vi "Calc Record Length.vi"(8 "error in (no error)":errorcluster, 11 "Modbus PLC in":refnum<class "Modbus PLC.lvclass">) -> (0 "error out":errorcluster, 3 "Modbus PLC out":refnum<class "Modbus PLC.lvclass">)   [LabVIEW 2023, in "Modbus PLC.lvlib" / "Modbus PLC.lvclass"]
uses:
  Modbus PLC.lvclass
  Modbus PLC.lvclass/Modbus PLC.ctl
panel:
  out "Array":i32[][](array[numeric])
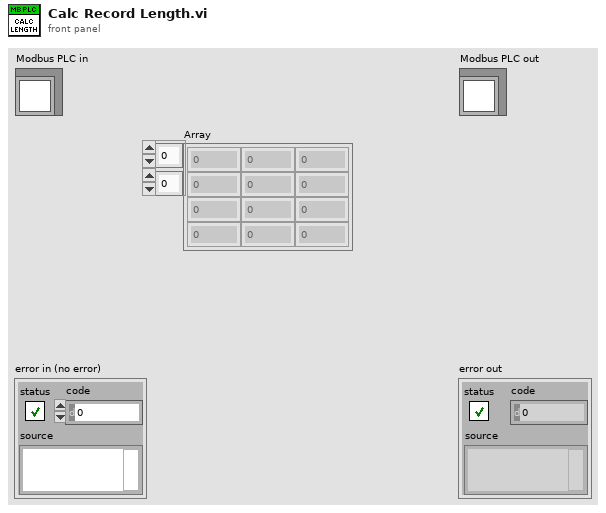
[diagram p1: front panel]
types:
  T1 = typedef "Modbus PLC.lvlib/Modbus PLC.lvclass/Input Map.ctl" = map{string, cluster{"Address":i32, "Data Type":enum16{"Int", "Float"}, "Reg Type":enum16{"Holding", "Input", "Coil"}}}
  T2 = typedef "Modbus PLC.lvlib/Modbus PLC.lvclass/Output Map.ctl" = map{string, cluster{"Address":i32, "Data Type":enum16{"Int", "Float"}, "Reg Type":enum16{"Holding", "Input", "Coil"}}}
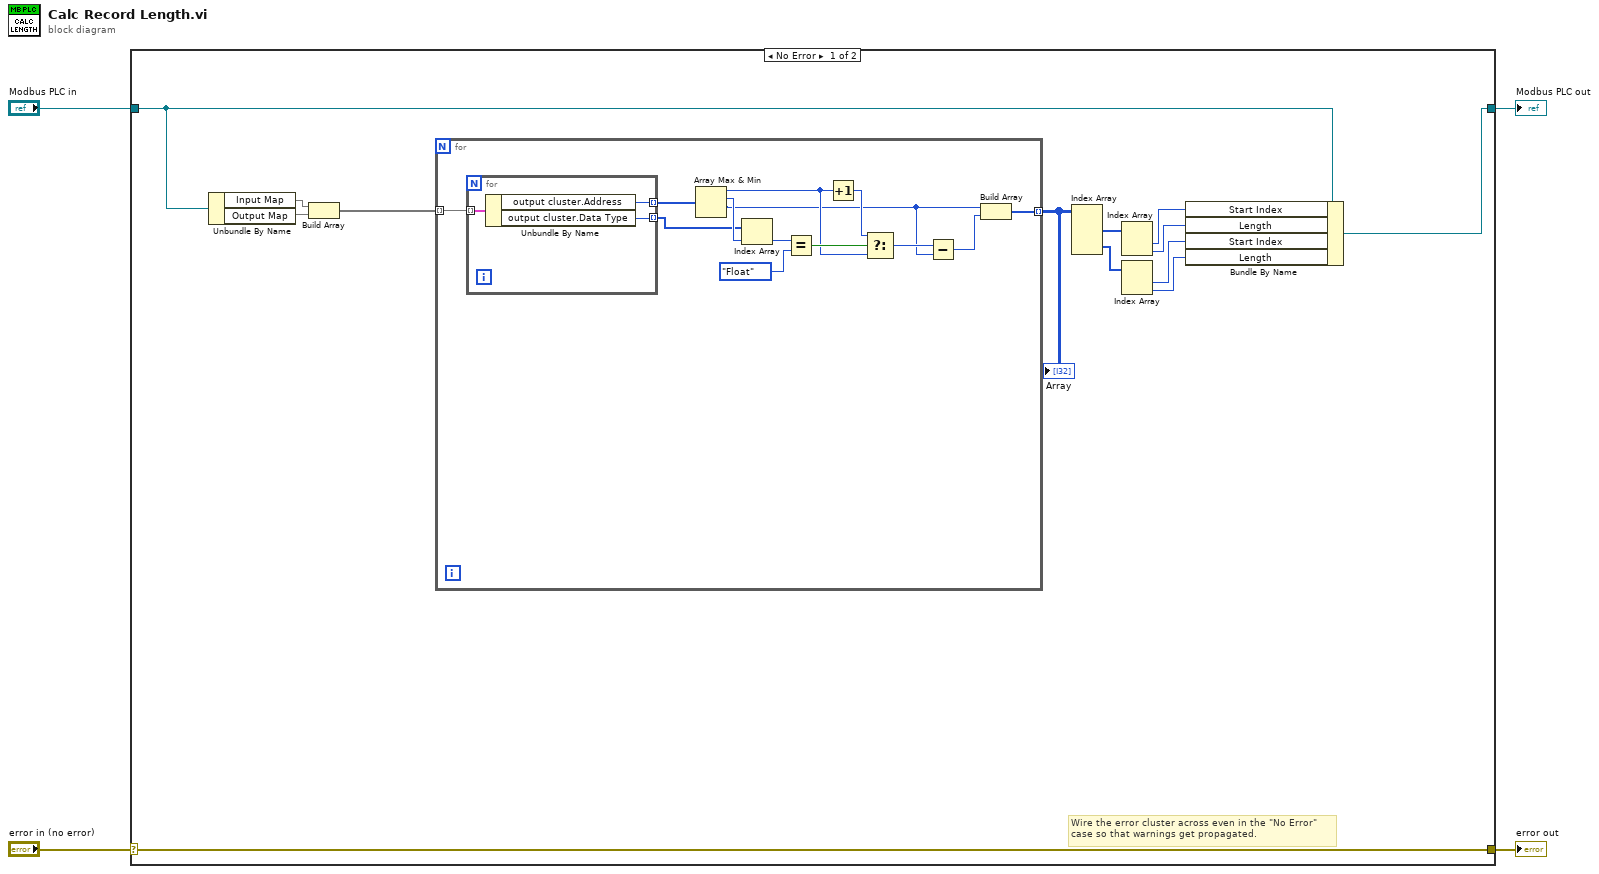
[diagram p0: block diagram]
diagram:
  n1 = case shown="No Error" "error in (no error)" {
    selector: "error in (no error)" -> [w17 w35]
    tunnel: [w17 w35] -> w3
    tunnel: [w5 w34] -> w1
    tunnel: "Modbus PLC in" -> [w13 w34]
    frame No Error {
      # "Wire the error cluster across even in the \"No Error\"\ncase so that warnings get propagated."
      n2 = Unbundle By Name(w13) -> ("Input Map"=w16:T1, "Output Map"=w15:T2)
      n3 = Build Array(w16, w15) -> (w14:T2[])
      n4 = for {
        tunnel: w14 -> [w30] mode=indexing
        tunnel: [w18] -> w12 mode=indexing
        n5 = for {
          tunnel: w30 -> [w33] mode=indexing
          tunnel: [w32] -> w29 mode=indexing
          tunnel: [w31] -> w27 mode=indexing
          n6 = Unbundle By Name(w33) -> ("output cluster.Address"=w32:i32, "output cluster.Data Type"=w31:enum16{"Int", "Float"})
        }
        n7 = Array Max & Min(array=w29) -> (max value=w22:i32, max index (indices)=w28:i32, min value=w20:i32)  [unwired: 1 out]
        n8 = Index Array(array=w27, index=w28) -> (element=w26:enum16{"Int", "Float"})
        n9 = Equal?(x=w26, y=enum16{"Int", "Float"}."Float") -> (x = y?=w24:bool)
        n10 = Increment(x=w22) -> (x+1=w23:i32)
        n11 = Select(t=w23, s=w24, f=w22) -> (s? t:f=w21:i32)
        n12 = Subtract(x=w21, y=w20) -> (x-y=w19:i32)
        n13 = Build Array(w20, w19) -> (w18:i32[])
      }
      "Array" <- w12
      n14 = Index Array(array=w12) -> (element #1=w11:i32[], element #2=w8:i32[])  [unwired: 4 in]
      n15 = Index Array(array=w11) -> (element #1=w10:i32, element #2=w9:i32)  [unwired: 2 in]
      n16 = Index Array(array=w8) -> (element #1=w7:i32, element #2=w6:i32)  [unwired: 2 in]
      n17 = Bundle By Name(cluster=w13, "Start Index"=w10, "Length"=w9, "Start Index"=w7, "Length"=w6) -> (w5:refnum<class "Modbus PLC.lvclass">)
    }
    frame Error {
    }
  }
  "error out" <- w3
  "Modbus PLC out" <- w1
